vi "Write Parent.vi"(8 "error in (no error)":errorcluster, 10 "parent":string, 11 "Asset Location in":refnum<class "Asset Location.lvclass">) -> (0 "error out":errorcluster, 3 "Asset Location out":refnum<class "Asset Location.lvclass">)   [LabVIEW 2019, in "Asset Location.lvclass"]
uses:
  Asset Location.lvclass
  Asset Location.lvclass/Asset Location.ctl
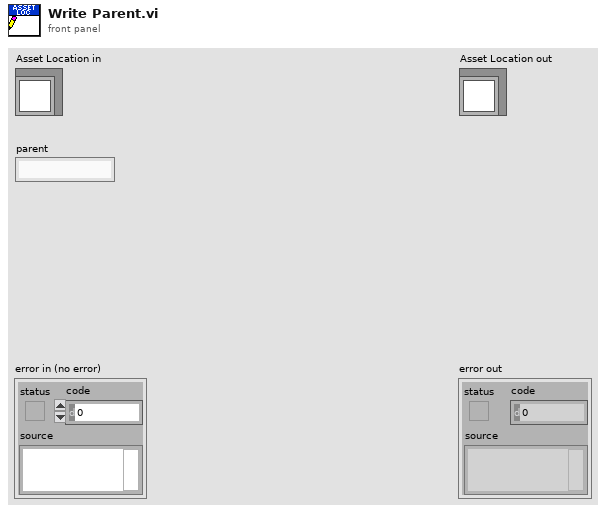
[diagram p1: front panel]
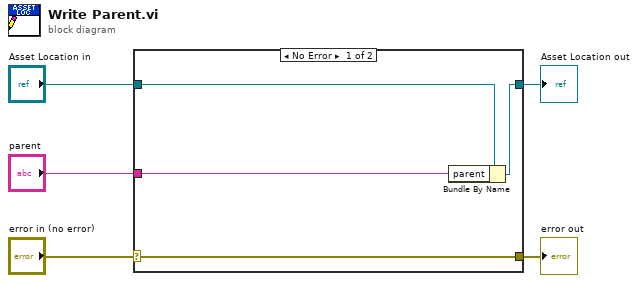
[diagram p0: block diagram]
diagram:
  n1 = case shown="No Error" "error in (no error)" {
    selector: "error in (no error)" -> [w9 w10]
    tunnel: [w9 w10] -> w4
    tunnel: [w7 w11] -> w2
    tunnel: "Asset Location in" -> [w8 w11]
    tunnel: "parent" -> [w6 _]
    frame No Error {
      n2 = Bundle By Name(cluster=w8, "parent"=w6) -> (w7:refnum<class "Asset Location.lvclass">)
    }
    frame Error {
    }
  }
  "error out" <- w4
  "Asset Location out" <- w2
